vi "DrawPoint3D.vi"(9 "Display":T1={"Mode"=enum."Inherit Value", "PointSize"=5.0, "LineWidth"=1.0}, 10 "Color":T2={"Alpha"=1.0, "Color"=16711680} {"Alpha" min=0.0 max=1.0 scale=0.0..1.0}, 11 "Points":T3[](array[typedef])) -> ()   [LabVIEW 2014]
uses:
  TypeDefs/Point3D.ctl
  TypeDefs/Color.ctl
  <vilib>/picture/3D Picture Control/Object/Create Object (name).vi
  <vilib>/picture/3D Picture Control/Object/Add Object (no reference).vi
  <vilib>/picture/3D Picture Control/NI_3D Picture Control.lvlib
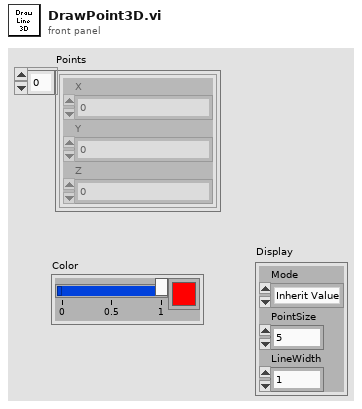
[diagram p1: front panel]
types:
  T1 = cluster{"Mode":enum16{"Inherit Value", "Points", "Wireframe", "Polygons"}, "PointSize":sgl, "LineWidth":sgl}
  T2 = typedef "Color.ctl" = cluster{"Alpha":dbl, "Color":u32}
  T3 = typedef "Point3D.ctl" = cluster{"X":sgl, "Y":sgl, "Z":sgl}
  T4 = enum16{"Points", "Lines", "Line Strip", "Line Loop", "Triangles", "Triangle Strip", "Triangle Fan", "Quads", "Quad Strip", "Polygon"}
  T5 = enum16{"New", "Find", "FindPattern", "GetTable", "Clear"}
  T6 = enum16{"Inherit Value", "Points", "Wireframe", "Polygons"}
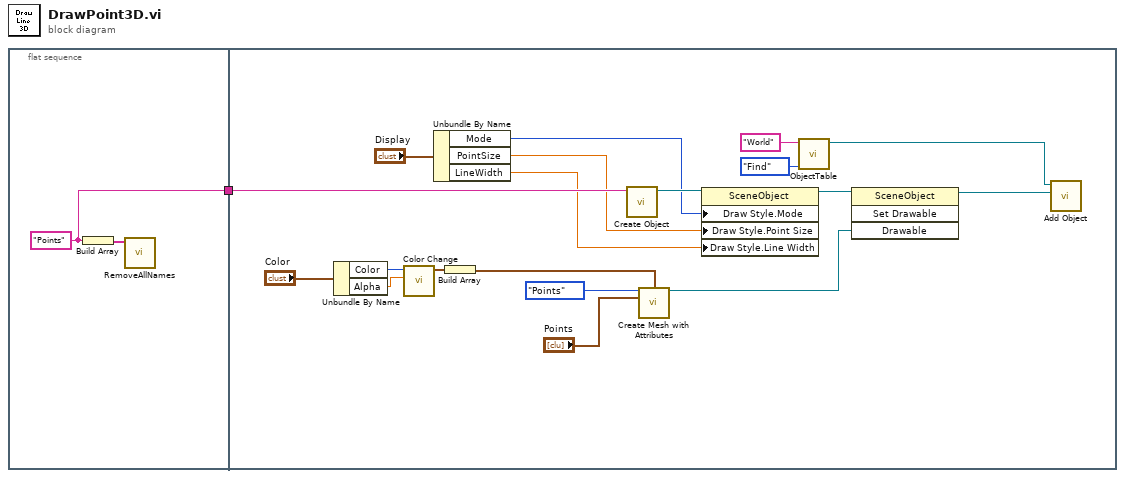
[diagram p0: block diagram]
diagram:
  n1 = flat-sequence {
    tunnel: [w2] -> w1
    tunnel: w1 -> [w9]
    frame #0 {
      w2 = "Points" ("string")
      n2 = Build Array(w2) -> (w3:string[])
      n3 = call "RemoveAllNames.vi"("Names"=w3) -> ()  [unwired: 11 in]
    }
    frame #1 {
      n4 = Unbundle By Name("Color") -> ("Color"=w15:u32, "Alpha"=w14:dbl)
      n5 = call <vilib>:"Color Change.vi"("Alpha"=w14, "Color"=w15) -> ("RGBA"=w16:cluster{"R":sgl, "G":sgl, "B":sgl, "A":sgl})  [unwired: 9 in]
      n6 = Unbundle By Name("Display") -> ("Mode"=w7:T6, "PointSize"=w6:sgl, "LineWidth"=w5:sgl)
      n7 = Build Array(w16) -> (w12:cluster{"R":sgl, "G":sgl, "B":sgl, "A":sgl}[])
      n8 = call-poly <vilib>:"Create Object.vi"("Name"=w9) -> ("Scene:New Object"=w11:refnum<vi>)  [unwired: 9 in, 1 out]
      n9 = call <vilib>:"Create Mesh with Attributes.vi"("Draw Mode"=T4."Points", "Color Array"=w12, "Vertex Array"="Points") -> ("New Mesh Refnum"=w17:refnum<vi>)  [unwired: 11 in, 1 out]
      n10 = property class="SceneObject"(reference=w11, "Draw Style.Mode"=w7, "Draw Style.Point Size"=w6, "Draw Style.Line Width"=w5) -> (reference out=w10:refnum<vi>)  [unwired: 1 in, 1 out]
      n11 = call "ObjectTable.vi"("ObjectStoreSelector"=T5."Find", "Name"="World") -> ("ObjectRef"=w18:refnum<vi>)  [unwired: 5 in, 4 out]
      n12 = invoke class="SceneObject" method="Set Drawable"(reference=w10, "Drawable"=w17) -> (reference out=w20:refnum<vi>)  [unwired: 2 in, 3 out]
      n13 = call-poly <vilib>:"Add Object.vi"("New Object In"=w20, "Scene Object In"=w18) -> ()  [unwired: 8 in, 2 out]
    }
  }
